vi "Swerve_Calculations.vi"() -> ()   [LabVIEW 2018]
panel:
  out "magnitude4":dbl
  out "magnitude3":dbl
  out "magnitude2":dbl
  out "magnitude1":dbl
  out "Wheel Angle4":dbl
  out "Wheel Angle3":dbl
  out "Wheel Angle2":dbl
  out "wheel angle 1":dbl
  in  "j1y":dbl
  in  "j1x":dbl
  in  "j2x":dbl
  in  "width":dbl
  in  "length":dbl
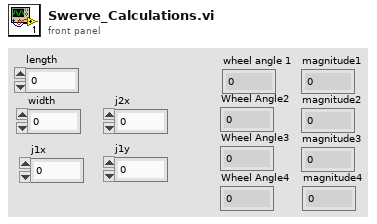
[diagram p1: front panel]
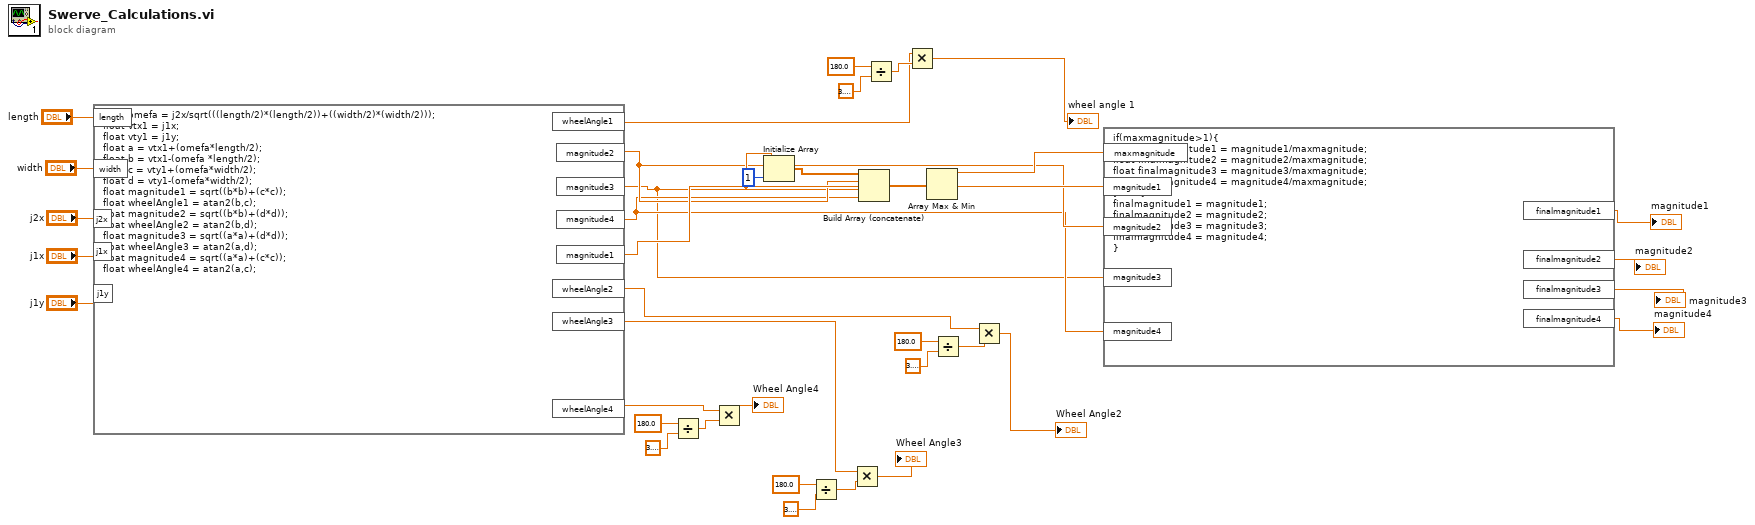
[diagram p0: block diagram]
diagram:
  n1 = formula code="float omefa = j2x/sqrt(((length/2)*(length/2))+((width/2)*(width/2)));\nfloat vtx1 = j1x;\nfloat vty1 = j1y;\nfloat a = vtx1+(omefa*length/2);\nfloat b = vtx1-(omefa *length/2);\nfloat c = vty1+(omefa*width/2);\nfloat d = vty1-(omefa*width/2);\nfloat magnitude1 = sqrt((b*b)+(c*c));\nfloat wheelAngle1 = atan2(b,c);\nfloat magnitude2 = sqrt((b*b)+(d*d));\nfloat wheelAngle2 = atan2(b,d);\nfloat magnitude3 = sqrt((a*a)+(d*d));\nfloat wheelAngle3 = atan2(a,d);\nfloat magnitude4 = sqrt((a*a)+(c*c));\nfloat wheelAngle4 = atan2(a,c);"("length"="length", "width"="width", "j2x"="j2x", "j1y"="j1y", "j1x"="j1x") -> ("wheelAngle1"=w7:dbl, "magnitude1"=w28:dbl, "magnitude2"=w27:dbl, "magnitude3"=w2:dbl, "magnitude4"=w26:dbl, "wheelAngle2"=w3:dbl, "wheelAngle3"=w15:dbl, "wheelAngle4"=w18:dbl)
  n2 = Divide(x=180.0, y=3.141592653589793) -> (x/y=w19:dbl)
  n3 = Multiply(x=w18, y=w19) -> (x*y=→"Wheel Angle4":dbl)
  n4 = Initialize Array(w28, 1 ("dimension size")) -> (w31:dbl[])
  n5 = Divide(x=180.0, y=3.141592653589793) -> (x/y=w14:dbl)
  n6 = Multiply(x=w15, y=w14) -> (x*y=→"Wheel Angle3":dbl)
  n7 = Build Array (concatenate)(w31, w27, w2, w26) -> (w30:dbl[])
  n8 = Divide(x=180.0, y=3.141592653589793) -> (x/y=w8:dbl)
  n9 = Multiply(x=w7, y=w8) -> (x*y=→"wheel angle 1":dbl)
  n10 = Array Max & Min(array=w30) -> (max value=w29:dbl)  [unwired: 3 out]
  n11 = Divide(x=180.0, y=3.141592653589793) -> (x/y=w1:dbl)
  n12 = Multiply(x=w3, y=w1) -> (x*y=→"Wheel Angle2":dbl)
  n13 = formula code="if(maxmagnitude>1){\nfloat finalmagnitude1 = magnitude1/maxmagnitude;\nfloat finalmagnitude2 = magnitude2/maxmagnitude;\nfloat finalmagnitude3 = magnitude3/maxmagnitude;\nfloat finalmagnitude4 = magnitude4/maxmagnitude;\n}else{\nfinalmagnitude1 = magnitude1;\nfinalmagnitude2 = magnitude2;\nfinalmagnitude3 = magnitude3;\nfinalmagnitude4 = magnitude4;\n}"("maxmagnitude"=w29, "magnitude2"=w27, "magnitude3"=w2, "magnitude4"=w26, "magnitude1"=w28) -> ("finalmagnitude1"=→"magnitude1":dbl, "finalmagnitude2"=→"magnitude2":dbl, "finalmagnitude3"=→"magnitude3":dbl, "finalmagnitude4"=→"magnitude4":dbl)
